vi "Cross Calibration 2.vi"(4 "RF data Out":T2={"Sampling Rate"=0, "Delay (micro s)"=0.5, "rf points per line"=500} {"Delay (micro s)" format="%.2f"}, 6 "Vert Settings":cluster{u16, i32, "Coupling":u16}, 8 "Motion Bd ID":T1=1 min=1 max=32 step=1) -> ()   [LabVIEW 2022 SP3]
uses:
  <instrlib>/Acqiris Dx/Acqiris Dx.lvlib
  ScanningControl/Motion Controllers/-MotionRoutines/MotionGlobals.vi
  <instrlib>/niScope/Acquire/Fetch/niScope Fetch.vi
  <vilib>/Utility/file.llb/Write To Spreadsheet File (string).vi
  <vilib>/Utility/file.llb/Write To Spreadsheet File (DBL).vi
  <vilib>/Analysis/NI_AAL_SigProc.lvlib
  <vilib>/Analysis/NI_AALBase.lvlib
  <vilib>/Analysis/baseanly.llb/Mean (DBL).vi
panel:
  out "Ch 1":dbl[][](graph)
  out "Ch 0":dbl[][](graph)
  out "Data Array":cluster{dbl[], dbl[], dbl[], dbl[]}
  in  "Attenuator":dbl=100.0
  in  "Num Voltage Steps":i32=20
  in  "Average":i32
  out "current f":dbl
  in  "Freq Step Size (MHz)":dbl=2.0 format="%.2f"
  in  "Start frequency (MHz)":dbl=1.0 format="%.2f"
  in  "Cal Tran":bool
  in  "Set up Digi":bool
  in  "ExitSendCmd":bool
  in  "Save":bool
  out "current V":dbl
  in  "Hydrophone 2":u16(ring) items=["Agilent", "Tabor"]
  in  "Voltage Step Size (mVpp)":dbl=10.0 format="%.2f"
  in  "Num Freq Steps":i32=20
  in  "Start voltage (mVpp)":dbl=50.0 format="%.3f"
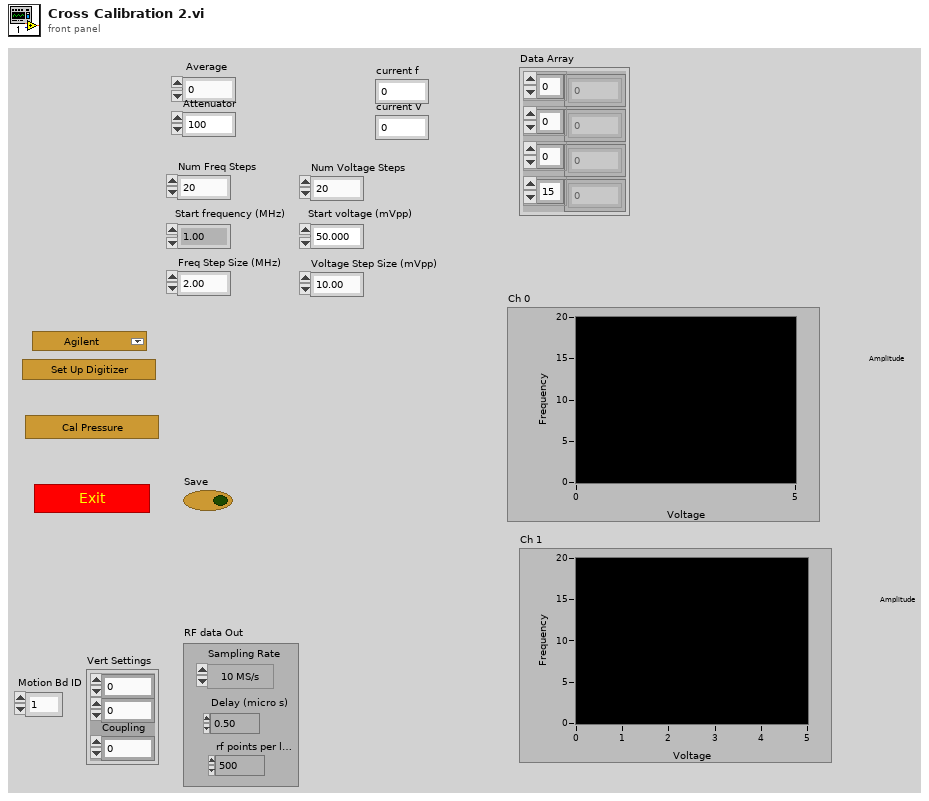
[diagram p1: front panel]
types:
  T1 = typedef "Board Id" = u8
  T2 = cluster{"Sampling Rate":u16, "Delay (micro s)":dbl, "rf points per line":u16}
  T3 = cluster{"Sampling Rate":dbl, "Ref Delay (ms)":dbl, "rf points per line":i32}
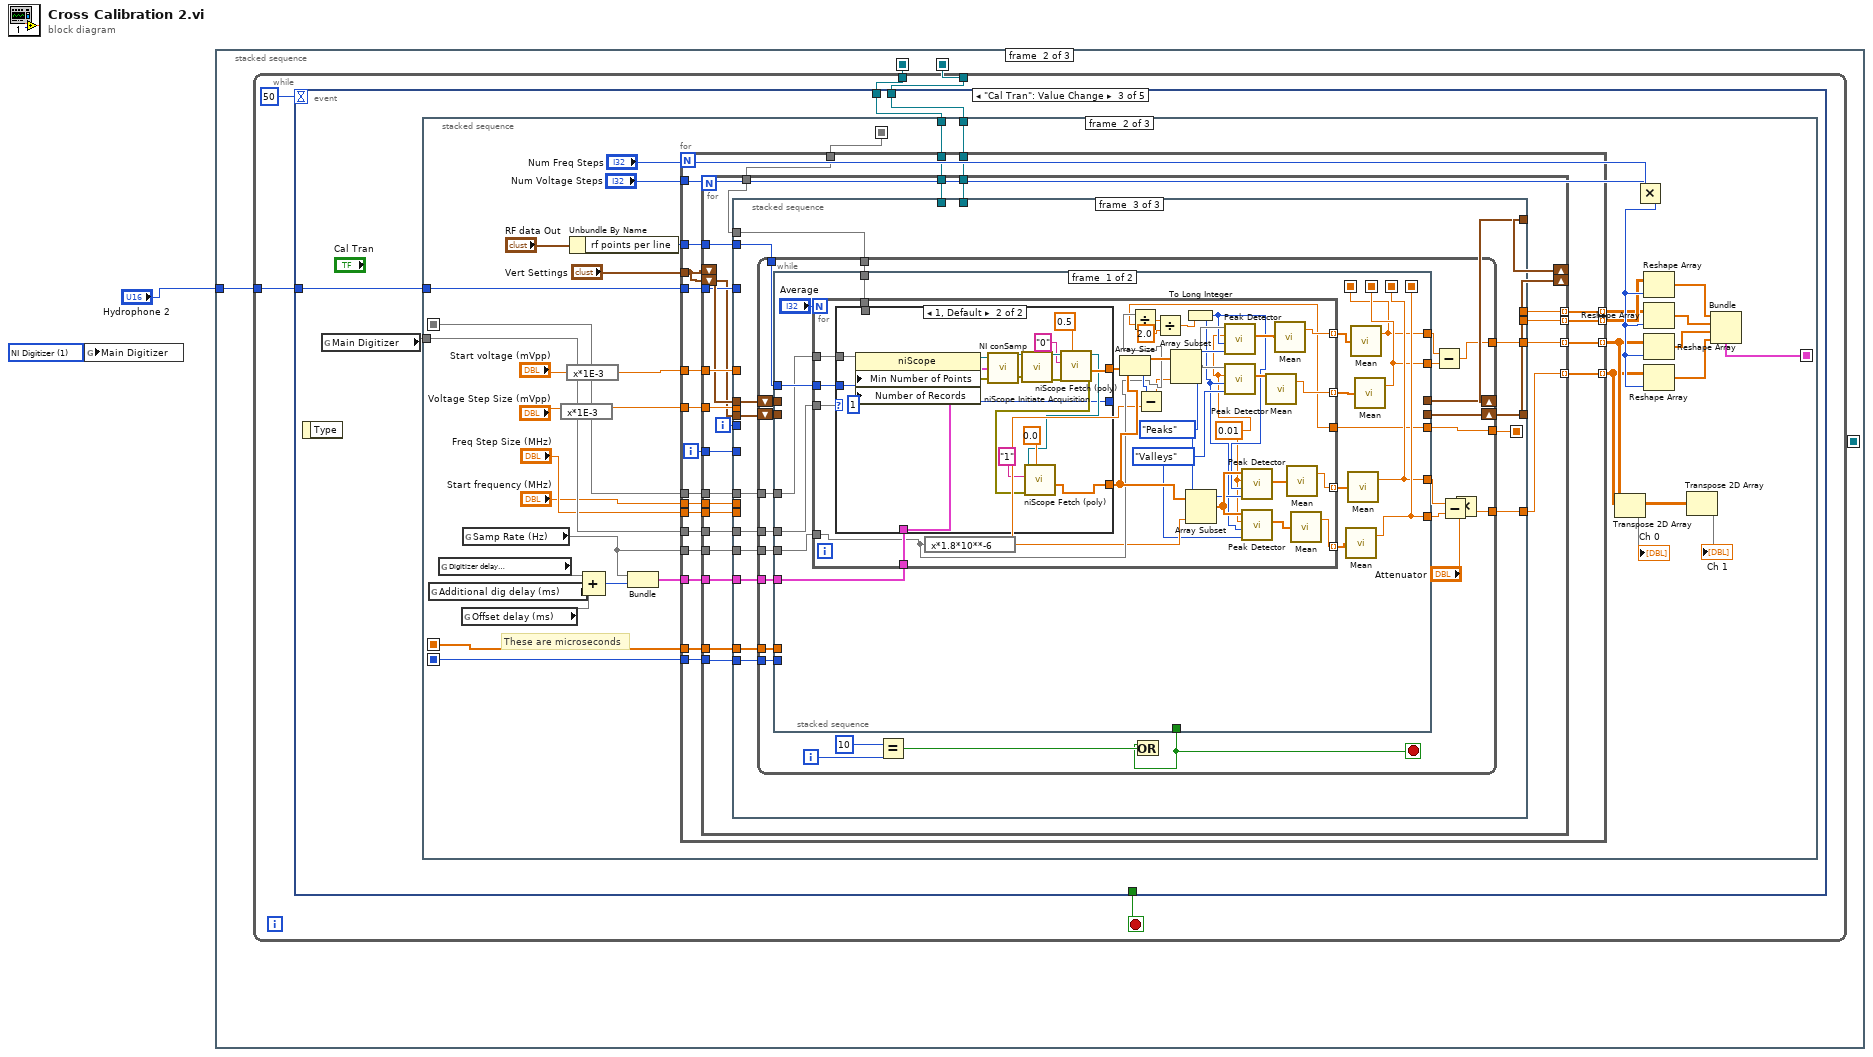
[diagram p0: block diagram]
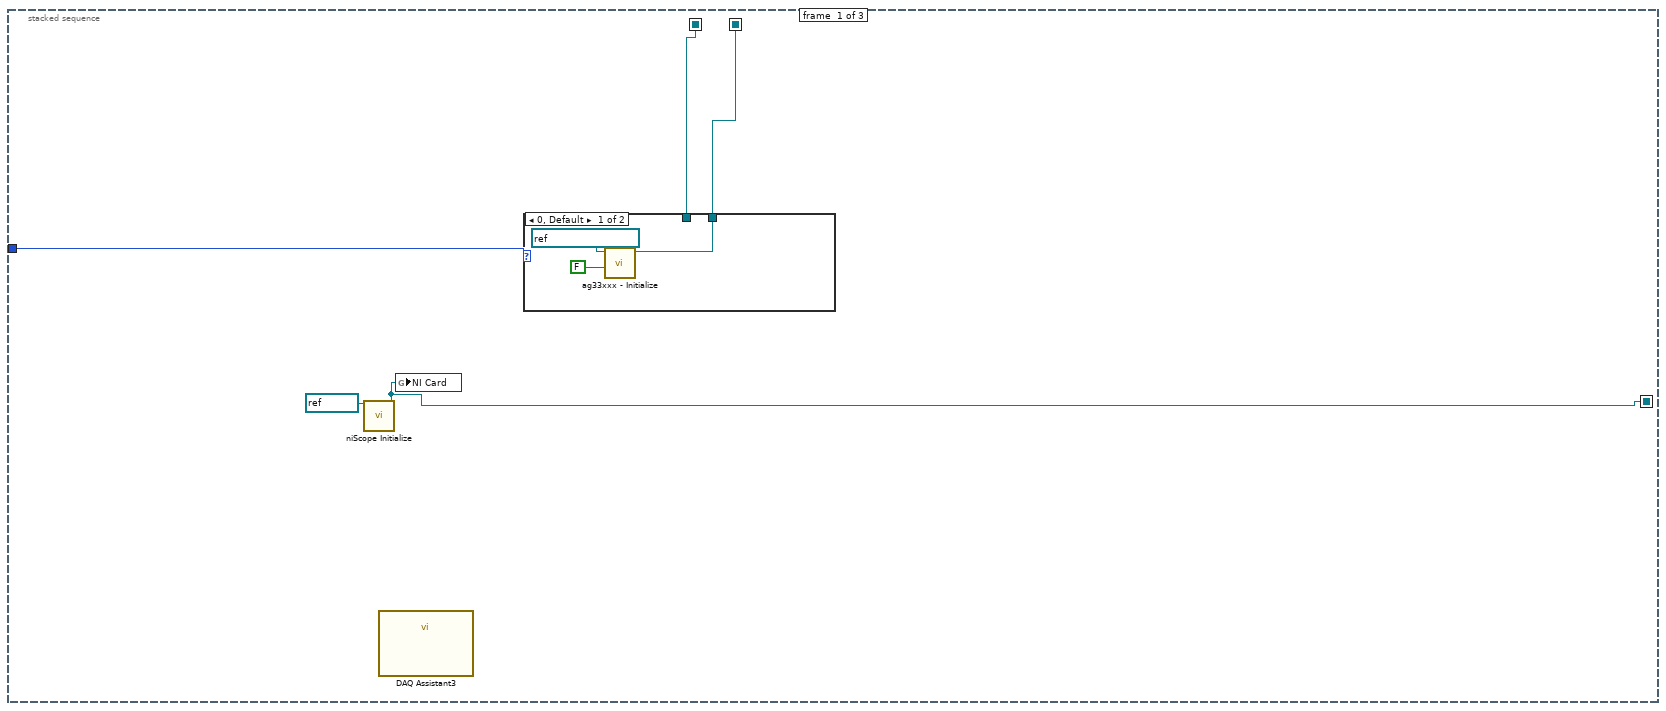
[diagram p2: hidden frame]
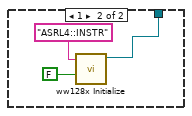
[diagram p3: hidden frame]
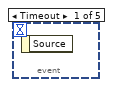
[diagram p4: hidden frame]
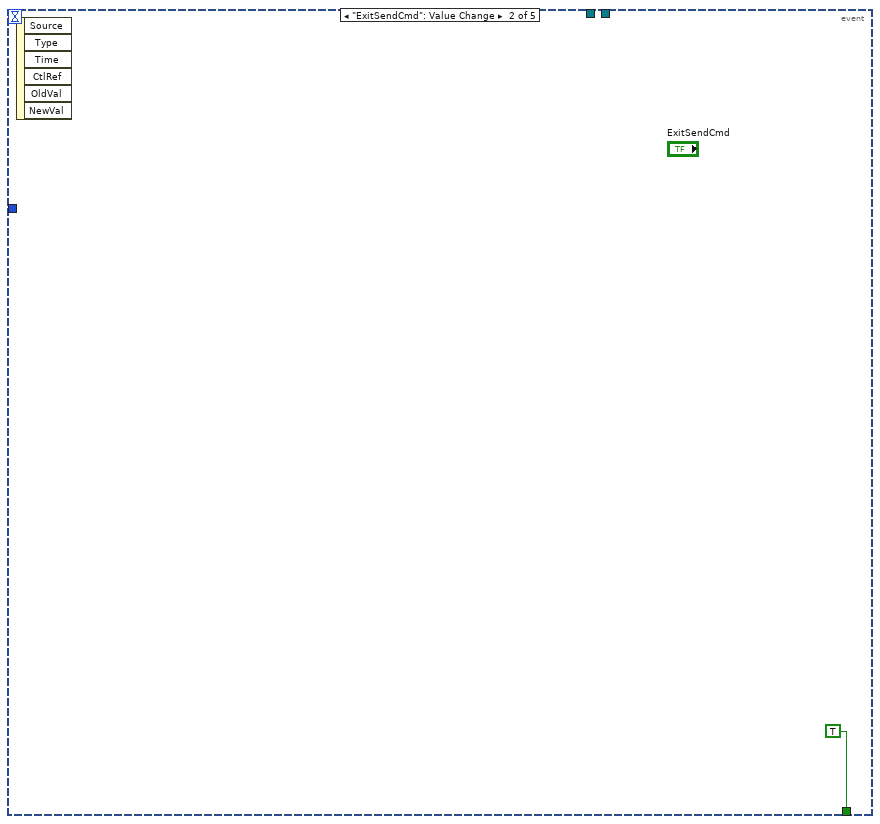
[diagram p5: hidden frame]
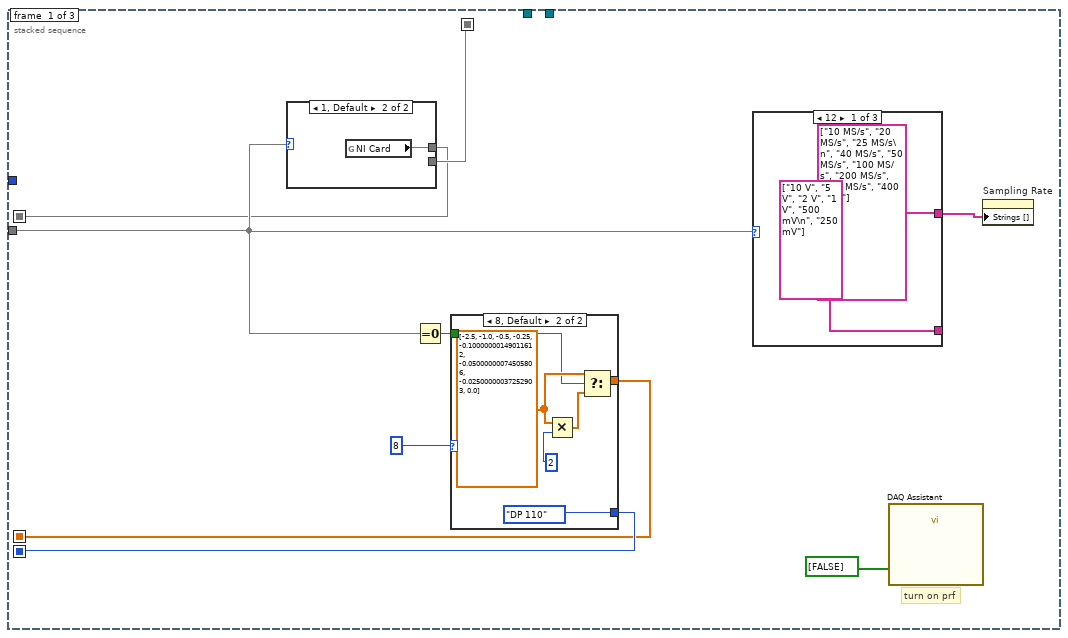
[diagram p6: hidden frame]
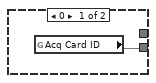
[diagram p7: hidden frame]
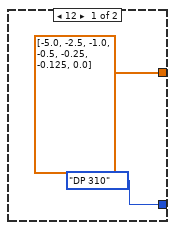
[diagram p8: hidden frame]
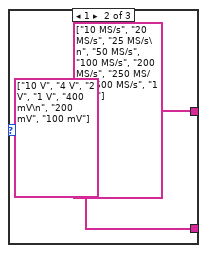
[diagram p9: hidden frame]
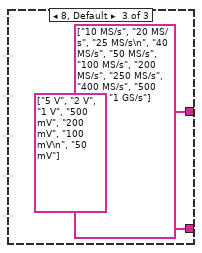
[diagram p10: hidden frame]
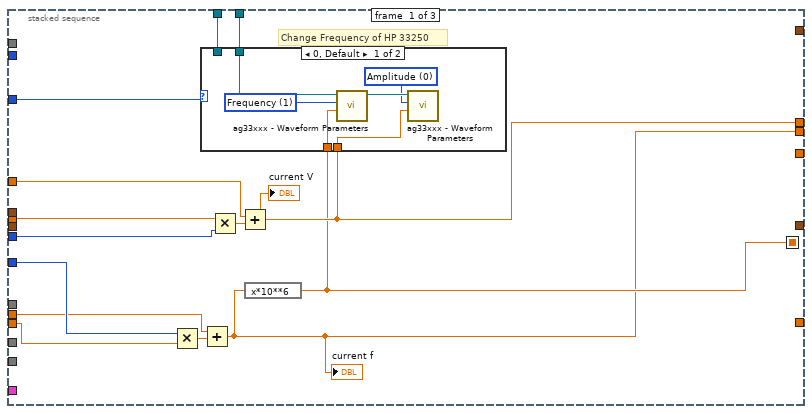
[diagram p11: hidden frame]
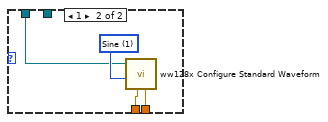
[diagram p12: hidden frame]
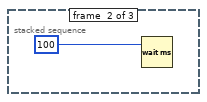
[diagram p13: hidden frame]
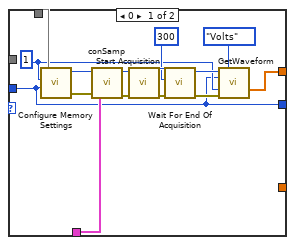
[diagram p14: hidden frame]
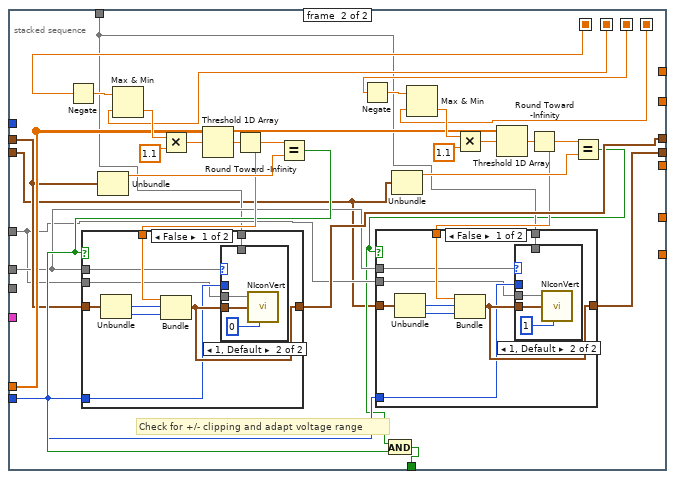
[diagram p15: hidden frame]
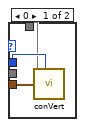
[diagram p16: hidden frame]
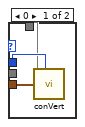
[diagram p18: hidden frame]
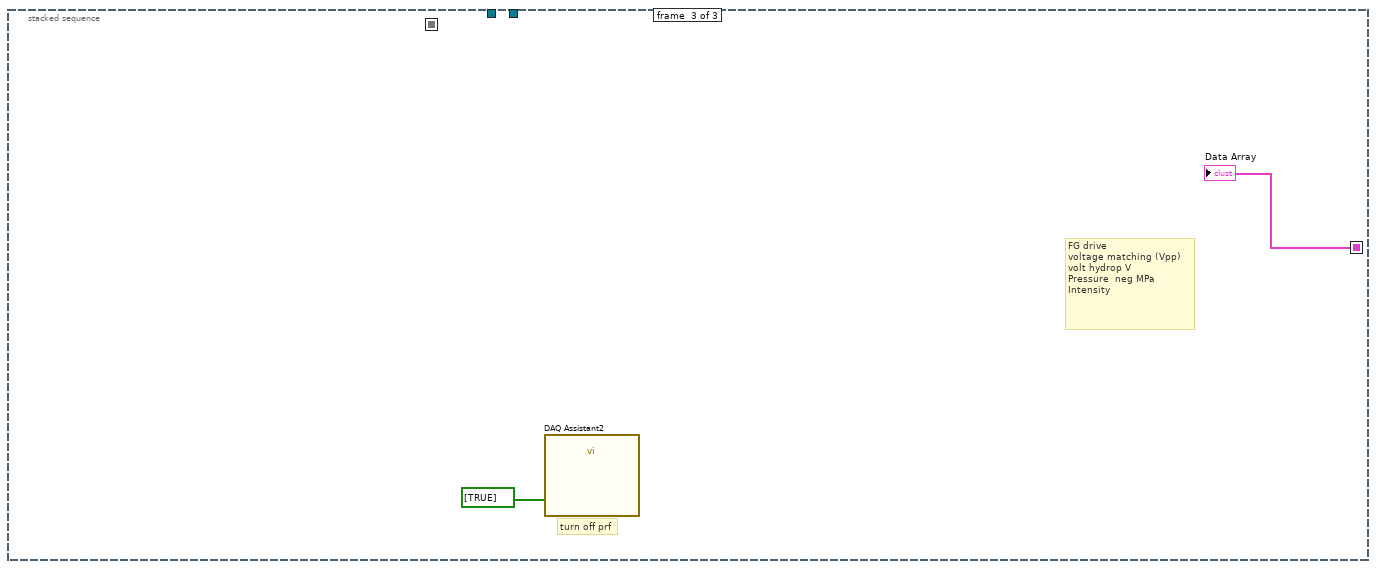
[diagram p20: hidden frame]
diagram:
  w1 = u16 1 items=["Acqiris Digitzer", "NI Digitizer"] ("Main Digitizer")
  n1 = global write "MotionGlobals.vi" "Main Digitizer"(w1) -> ()
  n2 = stacked-sequence {
    seq-local: [w5 _ _] -> [_ _ w364]
    seq-local: [w3 _ _] -> [_ w15 w362]
    seq-local: [w4 _ _] -> [_ w14 w361]
    tunnel: "Hydrophone 2" -> [w6 w16 w363]
    frame #0 {
      n3 = call <instrlib>:"niScope Initialize.vi"("resource name"=refnum<k15> "DIG3") -> ("instrument handle"=w5:refnum<k15>)  [unwired: 3 in, 11 out]
      n4 = call "DAQ Assistant3"() -> ()  [unwired: 17 in, 3 out]
      n5 = global write "MotionGlobals.vi" "NI Card"(w5) -> ()
      n6 = case shown="0, Default" w6 {
        tunnel: [w9 _] -> w4
        tunnel: [_ w11] -> w3
        frame 0, Default {
          n7 = call <instrlib>:"ag33xxx - Initialize.vi"("Reset (T: Reset)"=FALSE, "Instrument Resource Name"=refnum<visa-resource-name> "GPIB::13::INSTR") -> ("dup VISA session"=w9:refnum<visa-resource-name>)  [unwired: 8 in, 1 out]
        }
        frame 1 {
          n8 = call <instrlib>:"ww128x Initialize.vi"("reset device (Yes)"=FALSE ("reset device"), "resource name"="ASRL4::INSTR") -> ("instrument handle out"=w11:refnum<k15>)  [unwired: 2 in, 7 out]
        }
      }
    }
    frame #1 {
      n9 = while {
        tunnel: w16 -> [w19]
        tunnel: w15 -> [w18]
        tunnel: w14 -> [w17]
        stop <- w21 stop-if-true
        n10 = event shown="[2] \"Cal Tran\": Value Change" {
          selector: _ -> [_ _ _ _ _]
          dyn-events: _ -> [_ _ _ _ _]
          timeout: 50 -> [_ _ _ _ _]
          tunnel: [_ TRUE _ _ _] -> w21
          tunnel: w19 -> [_ _ w25 _ _]
          tunnel: w18 -> [_ _ w24 _ _]
          tunnel: w17 -> [_ _ w23 _ _]
          event Timeout {
            n11 = event-data() -> ()  [unwired: 2 out]
          }
          event "ExitSendCmd": Value Change {
            n12 = event-data() -> ()  [unwired: 7 out]
          }
          event "Cal Tran": Value Change {
            n13 = event-data() -> ()  [unwired: 2 out]
            n14 = global read "MotionGlobals.vi" "Main Digitizer"() -> (w26)
            n15 = stacked-sequence {
              seq-local: [w33 _ _] -> [_ w86 _]
              seq-local: [w34 _ _] -> [_ w87 _]
              seq-local: [w30 _ _] -> [_ w81 _]
              seq-local: [_ w72 _] -> [_ _ w341]
              seq-local: [w29 _ _] -> [_ w71 _]
              tunnel: w26 -> [w32 w80 _]
              tunnel: w25 -> [_ w70 _]
              tunnel: w24 -> [_ w69 _]
              tunnel: w23 -> [_ w68 _]
              frame #0 {
                # "turn on prf"
                n16 = case shown="1, Default" w32 {
                  tunnel: [w36 _] -> w30
                  tunnel: [_ w37] -> w29
                  frame 0 {
                    n17 = global read "MotionGlobals.vi" "Acq Card ID"() -> (w36)
                  }
                  frame 1, Default {
                    n18 = global read "MotionGlobals.vi" "NI Card"() -> (w37)
                  }
                }
                n19 = Equal To 0?(x=w32) -> (x = 0?=w35:bool)
                n20 = case shown="8, Default" 8 {
                  tunnel: [sgl[] [-5.0, -2.5, -1.0, -0.5, -0.25, -0.125, 0.0] w40] -> w33
                  tunnel: [enum16{"DP 110", "DP 310"}."DP 310" ("Card Type") enum16{"DP 110", "DP 310"}."DP 110" ("Card Type")] -> w34
                  tunnel: w35 -> [_ w41]
                  frame 12 {
                  }
                  frame 8, Default {
                    w42 = sgl[] [-2.5, -1.0, -0.5, -0.25, -0.1, -0.05, -0.025, 0.0]
                    n21 = Multiply(x=w42, y=2) -> (x*y=w43:sgl[])
                    n22 = Select(t=w42, s=w41, f=w43) -> (s? t:f=w40:sgl[])
                  }
                }
                n23 = case shown="12" w32 {
                  tunnel: [string[] ["10 MS/s", "20 MS/s", "25 MS/s\n", "40 MS/s", "50 MS/s", "100 MS/s", "200 MS/s", "250 MS/s", "400 MS/s"] ("Strings []") string[] ["10 MS/s", "20 MS/s", "25 MS/s\n", "50 MS/s", "100 MS/s", "200 MS/s", "250 MS/s", "500 MS/s", "1 GS/s"] ("Strings []") string[] ["10 MS/s", "20 MS/s", "25 MS/s\n", "40 MS/s", "50 MS/s", "100 MS/s", "200 MS/s", "250 MS/s", "400 MS/s", "500 MS/s", "1 GS/s"] ("Strings []")] -> w31
                  tunnel: [string[] ["10 V", "5 V", "2 V", "1 V", "500 mV\n", "250 mV"] ("Strings []") string[] ["10 V", "4 V", "2 V", "1 V", "400 mV\n", "200 mV", "100 mV"] ("Strings []") string[] ["5 V", "2 V", "1 V", "500 mV", "200 mV", "100 mV\n", "50 mV"] ("Strings []")] -> _
                  frame 12 {
                  }
                  frame 1 {
                  }
                  frame 8, Default {
                  }
                }
                n24 = call "DAQ Assistant"("data"=bool[] [FALSE]) -> ()  [unwired: 3 in, 16 out]
                n25 = property on="Sampling Rate" class="Ring (strict)"("Strings []"=w31) -> ()  [unwired: 2 in, 2 out]
              }
              frame #1 {
                # "These are microseconds"
                n26 = global read "MotionGlobals.vi" "Additional dig delay (ms)"() -> (w78)
                n27 = global read "MotionGlobals.vi" "Digitizer delay\n (ms)"() -> (w76)
                n28 = global read "MotionGlobals.vi" "Offset delay (ms)"() -> (w79)
                n29 = global read "MotionGlobals.vi" "Samp Rate (Hz)"() -> (w64)
                n30 = expression code="x*1E-3"("Voltage Step Size (mVpp)") -> (w84:dbl)
                n31 = expression code="x*1E-3"("Start voltage (mVpp)") -> (w82:dbl)
                n32 = Unbundle By Name("RF data Out") -> ("rf points per line"=w88:u16)
                n33 = Compound Arithmetic op=ADD(w76, w78, w79) -> (w77:i32)
                n34 = Bundle("Samp Rate (Hz)"=w64, w77) -> (w75:cluster{"Samp Rate (Hz)":void, i32})  [unwired: 1 out]
                n35 = for {
                  N: "Num Freq Steps" -> [_]
                  tunnel: "Num Voltage Steps" -> [w110]
                  tunnel: w88 -> [w109]
                  tunnel: w87 -> [w108]
                  tunnel: w86 -> [w107]
                  tunnel: w84 -> [w106]
                  tunnel: w82 -> [w105]
                  tunnel: w81 -> [w104]
                  tunnel: w80 -> [w103]
                  tunnel: w75 -> [w102]
                  tunnel: "Vert Settings" -> [w89]
                  tunnel: w71 -> [w101]
                  tunnel: w70 -> [w100]
                  tunnel: w69 -> [w99]
                  tunnel: w68 -> [w98]
                  tunnel: "Freq Step Size (MHz)" -> [w96]
                  tunnel: "Start frequency (MHz)" -> [w95]
                  tunnel: w64 -> [w94]
                  tunnel: [w93] -> w63 mode=indexing
                  tunnel: [w92] -> w56 mode=indexing
                  tunnel: [w91] -> w60 mode=indexing
                  tunnel: [w90] -> w59 mode=indexing
                  i -> [w97]
                  n36 = for {
                    N: w110 -> [_]
                    tunnel: w106 -> [w134]
                    tunnel: w105 -> [w133]
                    tunnel: w104 -> [w132]
                    tunnel: w109 -> [w131]
                    shift-right: [w130] -> _
                    shift-left: w89 -> [w129]
                    tunnel: w100 -> [w128]
                    tunnel: w107 -> [w127]
                    tunnel: w108 -> [w126]
                    tunnel: w103 -> [w125]
                    tunnel: w101 -> [w124]
                    tunnel: w102 -> [w123]
                    tunnel: w99 -> [w122]
                    tunnel: w98 -> [w121]
                    tunnel: w97 -> [w120]
                    tunnel: w96 -> [w119]
                    tunnel: w95 -> [w118]
                    tunnel: w94 -> [w117]
                    tunnel: [w116] -> w93 mode=indexing
                    tunnel: [w111] -> w92 mode=indexing
                    tunnel: [w115] -> w91 mode=indexing
                    tunnel: [w114] -> w90 mode=indexing
                    shift-right: [w113] -> _
                    shift-left: w89 -> [w112]
                    i -> [w135]
                    n37 = stacked-sequence {
                      seq-local: [w137 _ _] -> [_ _ w165]
                      tunnel: w135 -> [w149 _ _]
                      tunnel: w134 -> [w148 _ _]
                      tunnel: w133 -> [w147 _ _]
                      tunnel: w132 -> [_ _ w175]
                      tunnel: w131 -> [_ _ w173]
                      tunnel: w129 -> [_ _ w164]
                      tunnel: [_ _ w174] -> w130
                      tunnel: w128 -> [w146 _ _]
                      tunnel: w127 -> [_ _ w172]
                      tunnel: w126 -> [_ _ w171]
                      tunnel: w125 -> [_ _ w170]
                      tunnel: w124 -> [_ _ w169]
                      tunnel: w123 -> [_ _ w168]
                      tunnel: w122 -> [w145 _ _]
                      tunnel: w121 -> [w144 _ _]
                      tunnel: w120 -> [w141 _ _]
                      tunnel: w119 -> [w140 _ _]
                      tunnel: w118 -> [w139 _ _]
                      tunnel: w117 -> [_ _ w167]
                      tunnel: [_ _ w166] -> w116
                      tunnel: [_ _ w161] -> w111
                      tunnel: [w136 _ _] -> w115
                      tunnel: [w138 _ _] -> w114
                      tunnel: [_ _ w163] -> w113
                      tunnel: w112 -> [_ _ w162]
                      frame #0 {
                        # "Change Frequency of HP 33250"
                        n38 = Multiply(x=w141, y=w140) -> (x*y=w143:dbl)
                        n39 = Add(x=w139, y=w143) -> (x+y=w136:dbl)
                        "current f" <- w136
                        n40 = Multiply(x=w148, y=w149) -> (x*y=w142:dbl)
                        n41 = Add(x=w147, y=w142) -> (x+y=w138:dbl)
                        "current V" <- w138
                        n42 = expression code="x*10**6"(w136) -> (w137:dbl)
                        n43 = case shown="0, Default" w146 {
                          tunnel: w138 -> [w150 w159]
                          tunnel: w137 -> [w151 w157]
                          tunnel: w145 -> [_ w156]
                          tunnel: w144 -> [w155 _]
                          frame 0, Default {
                            w152 = u16 0 items=["Amplitude", "Frequency", "Offset"] ("Parameter (0: Amplitude)")
                            w153 = u16 1 items=["Amplitude", "Frequency", "Offset"] ("Parameter (0: Amplitude)")
                            n44 = call <instrlib>:"ag33xxx - Waveform Parameters.vi"("Value (1.00)"=w151, "Parameter (0: Amplitude)"=w153, "VISA session"=w155) -> ("dup VISA session"=w154:refnum<visa-resource-name>)  [unwired: 7 in, 1 out]
                            n45 = call <instrlib>:"ag33xxx - Waveform Parameters.vi"("Value (1.00)"=w150, "Parameter (0: Amplitude)"=w152, "VISA session"=w154) -> ()  [unwired: 7 in, 2 out]
                          }
                          frame 1 {
                            w158 = 1 items=["Sine"=1, "Square"=2, "Triangle"=3, "Ramp Up"=4, "Ramp Down"=5, "DC"=6, "Ramp"=1001, "Pulse"=1005, "Sync"=1002, "Gaussian"=1003, "Exponential"=1004, "Noise"=1006] ("waveform")
                            n46 = call <instrlib>:"ww128x Configure Standard Waveform.vi"("amplitude"=w159, "frequency"=w157, "waveform"=w158, "instrument handle"=w156) -> ()  [unwired: 4 in, 4 out]
                          }
                        }
                      }
                      frame #1 {
                        n47 = Wait (ms)(milliseconds to wait=100) -> ()  [unwired: 1 out]
                      }
                      frame #2 {
                        n48 = while {
                          tunnel: w175 -> [w200]
                          shift-right: [w199] -> w174
                          shift-left: w164 -> [w198]
                          tunnel: w173 -> [w197]
                          tunnel: w172 -> [w196]
                          tunnel: w171 -> [w195]
                          tunnel: w170 -> [w191]
                          tunnel: w169 -> [w190]
                          tunnel: w168 -> [w189]
                          tunnel: w167 -> [w188]
                          tunnel: [w183] -> w166
                          tunnel: [w177] -> w161
                          tunnel: w165 -> [w181]
                          shift-right: [w179] -> w163
                          shift-left: w162 -> [w178]
                          i -> [w194]
                          stop <- w180 stop-if-true
                          n49 = stacked-sequence {
                            seq-local: [w203 _] -> [_ w300]
                            seq-local: [w202 _] -> [_ w301]
                            seq-local: [w204 _] -> [_ w290]
                            seq-local: [w205 _] -> [_ w289]
                            tunnel: w200 -> [w216 w283]
                            tunnel: [_ w299] -> w199
                            tunnel: w198 -> [_ w287]
                            tunnel: w197 -> [w215 _]
                            tunnel: w196 -> [_ w288]
                            tunnel: w195 -> [_ w284]
                            tunnel: [_ w281] -> w180
                            tunnel: w191 -> [w214 w286]
                            tunnel: w190 -> [w213 w285]
                            tunnel: w189 -> [w212 _]
                            tunnel: w188 -> [w210 _]
                            tunnel: [w205 _] -> w187
                            tunnel: [w204 _] -> w186
                            tunnel: [w203 _] -> w185
                            tunnel: [w202 _] -> w184
                            tunnel: w181 -> [w201 _]
                            tunnel: [_ w280] -> w179
                            tunnel: w178 -> [_ w279]
                            frame #0 {
                              n50 = for {
                                N: "Average" -> [_]
                                tunnel: w216 -> [w245]
                                tunnel: w215 -> [w244]
                                tunnel: w214 -> [w243]
                                tunnel: w213 -> [w242]
                                tunnel: w212 -> [w241]
                                tunnel: w210 -> [w227]
                                tunnel: [w231] -> w209 mode=indexing
                                tunnel: [w230] -> w208 mode=indexing
                                tunnel: [w229] -> w207 mode=indexing
                                tunnel: [w228] -> w206 mode=indexing
                                tunnel: w201 -> [w224]
                                w217 = 0.01 ("threshold")
                                w221 = enum32{"Peaks", "Valleys"}."Valleys" ("peaks/valleys")
                                w235 = enum32{"Peaks", "Valleys"}."Peaks" ("peaks/valleys")
                                n51 = case shown="1, Default" w243 {
                                tunnel: w245 -> [w254 _]
                                tunnel: w244 -> [w246 w262]
                                tunnel: [w252 w276] -> w240
                                tunnel: w242 -> [_ w274]
                                tunnel: w241 -> [w247 w268]
                                tunnel: [_ w261] -> w239
                                tunnel: [w246 w262] -> _
                                frame 0 {
                                w253 = 1
                                n52 = call <instrlib>:"Configure Memory Settings.vi"("Number of Samples (1000)"=w246, "Number of Segments (1)"=w253, "Instrument ID"=w254) -> ("error out"=w248:errorcluster, "dup Instrument ID"=w251:u32)  [unwired: 1 in, 2 out]
                                n53 = call "conSamp.vi"("error in"=w248, "Sampling"=w247, "InstrumentID"=w251) -> ("error out"=w249:errorcluster, "DUP ID"=w250:u32)
                                n54 = call <instrlib>:"Start Acquisition.vi"("error in (no error)"=w249, "Instrument ID"=w250) -> ("error out"=w258:errorcluster, "dup Instrument ID"=w259:u32)  [unwired: 2 in]
                                n55 = call <instrlib>:"Wait For End Of Acquisition.vi"("error in (no error)"=w258, "Timeout"=300, "Instrument ID"=w259) -> ("error out"=w256:errorcluster, "dup Instrument ID"=w257:u32)  [unwired: 3 out]
                                n56 = call "GetWaveform.vi"("Acq ID Out"=w257, "Read Mode"=enum32{"ADC", "Volts"}."Volts", "Num Samps"=w246, "Num Segs"=w253, "error in"=w256) -> ("first row"=w252:dbl[])  [unwired: 1 in, 9 out]
                                }
                                frame 1, Default {
                                n57 = property class="niScope"(reference=w274, "Min Number of Points"=w262, "Number of Records"=1) -> (reference out=w270:refnum<k15>, error out=w269:errorcluster)  [unwired: 1 in]
                                n58 = call "NI conSamp.vi"("error in"=w269, "Sampling"=w268, "InstrumentID"=w270) -> ("error out"=w271:errorcluster, "DUP ID"=w272:refnum<k15>)
                                n59 = call <instrlib>:"niScope Initiate Acquisition.vi"("instrument handle"=w272, "error in"=w271) -> ("instrument handle out"=w277:refnum<k15>, "error out"=w278:errorcluster)  [unwired: 12 out]
                                n60 = call-poly <instrlib>:"niScope Fetch (poly).vi"("timeout"=0.5, "error in"=w278, "channels"="0", "instrument handle"=w277) -> ("error out"=w265:errorcluster, "wfm"=w276:dbl[], "instrument handle out"=w263:refnum<k15>)  [unwired: 1 in, 4 out]
                                n61 = call-poly <instrlib>:"niScope Fetch (poly).vi"("timeout"=0.0, "error in"=w265, "channels"="1", "instrument handle"=w263) -> ("wfm"=w261:dbl[])  [unwired: 1 in, 6 out]
                                }
                                }
                                n62 = expression code="x*1.8*10**-6"(w227) -> (w223:dbl)
                                n63 = Array Size(array=w239) -> (size(s)=w238:i32)
                                n64 = Divide(x=w227, y=w224) -> (x/y=w226:dbl)
                                n65 = Subtract(x=w238, y=w223) -> (x-y=w222:dbl)
                                n66 = Divide(x=w226, y=2.0) -> (x/y=w219:dbl)
                                n67 = Array Subset(array=w240, length=w222) -> (w237:dbl[])  [unwired: 1 in]
                                n68 = To Long Integer(number=w219) -> (32bit integer=w218:i32)
                                n69 = Array Subset(array=w239, length=w223) -> (w236:dbl[])  [unwired: 1 in]
                                n70 = call <vilib>:"Peak Detector.vi"("peaks/valleys"=w235, "width"=w218, "threshold"=w217, "X"=w237) -> ("Amplitudes"=w234:dbl[])  [unwired: 3 in, 4 out]
                                n71 = call <vilib>:"Peak Detector.vi"("peaks/valleys"=w221, "width"=w218, "threshold"=w217, "X"=w237) -> ("Amplitudes"=w233:dbl[])  [unwired: 3 in, 4 out]
                                n72 = call <vilib>:"Peak Detector.vi"("peaks/valleys"=w235, "width"=w218, "threshold"=w217, "X"=w236) -> ("Amplitudes"=w232:dbl[])  [unwired: 3 in, 4 out]
                                n73 = call <vilib>:"Peak Detector.vi"("peaks/valleys"=w221, "width"=w218, "threshold"=w217, "X"=w236) -> ("Amplitudes"=w220:dbl[])  [unwired: 3 in, 4 out]
                                n74 = call-poly <vilib>:"Mean.vi"("X"=w233) -> ("mean"=w229:dbl)  [unwired: 1 out]
                                n75 = call-poly <vilib>:"Mean.vi"("X"=w234) -> ("mean"=w228:dbl)  [unwired: 1 out]
                                n76 = call-poly <vilib>:"Mean.vi"("X"=w232) -> ("mean"=w230:dbl)  [unwired: 1 out]
                                n77 = call-poly <vilib>:"Mean.vi"("X"=w220) -> ("mean"=w231:dbl)  [unwired: 1 out]
                              }
                              n78 = call-poly <vilib>:"Mean.vi"("X"=w209) -> ("mean"=w205:dbl)  [unwired: 1 out]
                              n79 = call-poly <vilib>:"Mean.vi"("X"=w208) -> ("mean"=w204:dbl)  [unwired: 1 out]
                              n80 = call-poly <vilib>:"Mean.vi"("X"=w206) -> ("mean"=w202:dbl)  [unwired: 1 out]
                              n81 = call-poly <vilib>:"Mean.vi"("X"=w207) -> ("mean"=w203:dbl)  [unwired: 1 out]
                            }
                            frame #1 {
                              # "Check for +/- clipping and adapt voltage range"
                              n82 = Negate(x=w301) -> (-x=w308:dbl)
                              n83 = Unbundle(w287) -> (w304:sgl)  [unwired: 2 out]
                              n84 = Max & Min(x=w308, y=w300) -> (min(x,y)=w306:dbl)  [unwired: 1 out]
                              n85 = Multiply(x=w306, y=1.1) -> (x*y=w307:dbl)
                              n86 = Threshold 1D Array(2:w307, 3:w288) -> (0:w303:sgl)  [unwired: 1 out]
                              n87 = Round Toward -Infinity(1:w303) -> (0:w302:sgl)
                              n88 = Equal?(x=w302, y=w304) -> (x = y?=w298:bool)
                              n89 = case shown="False" w298 {
                                tunnel: [w329 w340] -> w299
                                tunnel: w287 -> [w331 w340]
                                tunnel: w302 -> [w330 _]
                                tunnel: w284 -> [w328 _]
                                tunnel: w283 -> [w327 _]
                                tunnel: w286 -> [w326 _]
                                tunnel: w285 -> [w325 _]
                                frame False {
                                n90 = Unbundle(w331) -> (w333:i32, "Coupling"=w332:u16)  [unwired: 1 out]
                                n91 = Bundle(w330, w333, "Coupling"=w332) -> (w329:cluster{sgl, i32, "Coupling":u16})  [unwired: 1 out]
                                n92 = case shown="1, Default" w326 {
                                tunnel: w329 -> [w336 w339]
                                tunnel: w328 -> [w335 _]
                                tunnel: w327 -> [w334 _]
                                tunnel: w325 -> [_ w338]
                                frame 0 {
                                n93 = call "conVert.vi"("InstrumentID"=w334, 1:w335, "V scale"=w336) -> ()  [unwired: 2 in, 3 out]
                                }
                                frame 1, Default {
                                n94 = call "NIconVert.vi"("InstrumentID"=w338, "V scale"=w339, "Channel (0)"=0) -> ()  [unwired: 1 in, 4 out]
                                }
                                }
                                }
                                frame True {
                                }
                              }
                              n95 = Negate(x=w290) -> (-x=w297:dbl)
                              n96 = Unbundle(w279) -> (w293:sgl)  [unwired: 2 out]
                              n97 = Max & Min(x=w297, y=w289) -> (min(x,y)=w295:dbl)  [unwired: 1 out]
                              n98 = Multiply(x=w295, y=1.1) -> (x*y=w296:dbl)
                              n99 = Threshold 1D Array(2:w296, 3:w288) -> (0:w292:sgl)  [unwired: 1 out]
                              n100 = Round Toward -Infinity(1:w292) -> (0:w291:sgl)
                              n101 = Equal?(x=w291, y=w293) -> (x = y?=w282:bool)
                              n102 = case shown="False" w282 {
                                tunnel: [w313 w324] -> w280
                                tunnel: w279 -> [w315 w324]
                                tunnel: w291 -> [w314 _]
                                tunnel: w284 -> [w312 _]
                                tunnel: w283 -> [w311 _]
                                tunnel: w286 -> [w310 _]
                                tunnel: w285 -> [w309 _]
                                frame False {
                                n103 = Unbundle(w315) -> (w317:i32, "Coupling"=w316:u16)  [unwired: 1 out]
                                n104 = Bundle(w314, w317, "Coupling"=w316) -> (w313:cluster{sgl, i32, "Coupling":u16})  [unwired: 1 out]
                                n105 = case shown="1, Default" w310 {
                                tunnel: w313 -> [w320 w323]
                                tunnel: w312 -> [w319 _]
                                tunnel: w311 -> [w318 _]
                                tunnel: w309 -> [_ w322]
                                frame 0 {
                                n106 = call "conVert.vi"("InstrumentID"=w318, 1:w319, "V scale"=w320) -> ()  [unwired: 2 in, 3 out]
                                }
                                frame 1, Default {
                                n107 = call "NIconVert.vi"("InstrumentID"=w322, "V scale"=w323, "Channel (0)"=1) -> ()  [unwired: 1 in, 4 out]
                                }
                                }
                                }
                                frame True {
                                }
                              }
                              n108 = And(x=w282, y=w298) -> (x .and. y?=w281:bool)
                            }
                          }
                          n109 = Equal?(x=10, y=w194) -> (x = y?=w192:bool)
                          n110 = Or(x=w180, y=w192) -> ()  [unwired: 1 out]
                          n111 = Subtract(x=w184, y=w185) -> (x-y=w183:dbl)
                          n112 = Subtract(x=w186, y=w187) -> (x-y=w182:dbl)
                          n113 = Multiply(x="Attenuator", y=w182) -> (x*y=w177:dbl)
                        }
                      }
                    }
                  }
                }
                n114 = Transpose 2D Array(2D array=w63) -> (transposed array=→"Ch 0":dbl[][])
                n115 = Multiply(x="Num Freq Steps", y="Num Voltage Steps") -> (x*y=w65:i32)
                n116 = Reshape Array(w60, w65) -> (w58:dbl[])
                n117 = Reshape Array(w59, w65) -> (w57:dbl[])
                n118 = Reshape Array(w63, w65) -> (w61:dbl[])
                n119 = Reshape Array(w56, w65) -> (w62:dbl[])
                n120 = Transpose 2D Array(2D array=w56) -> (transposed array=→"Ch 1":dbl[][])
                n121 = Bundle(w58, w57, w61, w62) -> (w72:cluster{dbl[], dbl[], dbl[], dbl[]})  [unwired: 1 out]
              }
              frame #2 {
                # "turn off prf"
                # "FG drive\nvoltage matching (Vpp)\nvolt hydrop V\nPressure  neg MPa\nIntensity"
                n122 = call "DAQ Assistant2"("data"=bool[] [TRUE]) -> ()  [unwired: 3 in, 16 out]
                "Data Array" <- w341
              }
            }
          }
          event "Save": Value Change {
            n123 = event-data() -> ()  [unwired: 7 out]
            n124 = local read "Data Array"() -> (w348:cluster{dbl[], dbl[], dbl[], dbl[]})
            n125 = Build Array("Freq", "Voltage" ("element"), "Hydrophone Pk-Pk" ("element"), "Transducer Applied Voltage Pk-Pk" ("element")) -> (w353:string[])
            n126 = Unbundle(w348) -> (w347:dbl[], w346:dbl[], w345:dbl[], w344:dbl[])
            n127 = Build Array(w347, w346, w345, w344) -> (w343:dbl[][])
            n128 = call-poly <vilib>:"Write To Spreadsheet File.vi"("1D data"=w353) -> ("new file path (Not A Path if cancelled)"=w355:path)  [unwired: 5 in, 2 out]
            n129 = call-poly <vilib>:"Write To Spreadsheet File.vi"("transpose? (no:F)"=TRUE, "append to file? (new file:F)"=TRUE, "2D data"=w343, "file path (dialog if empty)"=w355) -> ()  [unwired: 2 in, 3 out]
          }
          event "Set up Digi": Value Change {
            n130 = event-data() -> ()  [unwired: 2 out]
            n131 = call "SetUpDigi.vi"("Motion Settings Out"="Motion Bd ID", "Therapy (T)"=TRUE) -> ("RF data Sampling Out"=w360:T3, "Vert Settings"=w359:cluster{dbl, dbl, "Coupling":u16})  [unwired: 3 in, 5 out]
            n132 = local write "Vert Settings"(w359) -> ()
            n133 = local write "RF data Out"(w360) -> ()
          }
        }
      }
    }
    frame #2 {
      n134 = case shown="0, Default" w363 {
        tunnel: w362 -> [_ w366]
        tunnel: w361 -> [w365 _]
        frame 0, Default {
          n135 = call <instrlib>:"ag33xxx - Close.vi"("VISA session"=w365) -> ()  [unwired: 10 in, 1 out]
        }
        frame 1 {
          n136 = call <instrlib>:"ww128x Close.vi"("instrument handle"=w366) -> ()  [unwired: 1 in, 10 out]
        }
      }
      n137 = call <instrlib>:"niScope Close.vi"("instrument handle"=w364) -> ()  [unwired: 1 in, 14 out]
    }
  }
